vi "get_config_multiplex.vi"(10 "target R":dbl format="%#_13g", 11 "configs":cluster{"R":dbl, "relays":bool[]}[](array[cluster])) -> (2 "index":i32, 3 "multiplexor":bool[](array[boolean]))   [LabVIEW 2018]
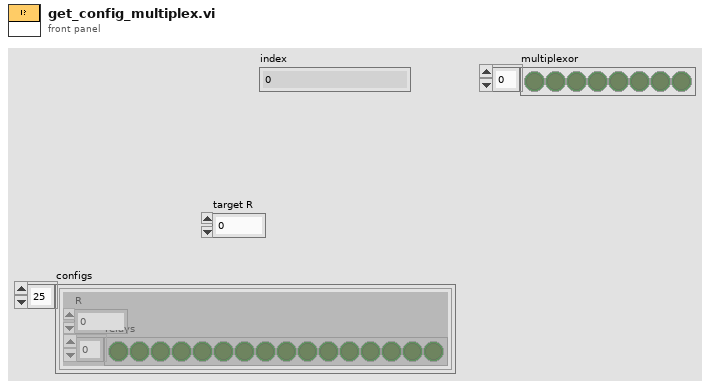
[diagram p1: front panel]
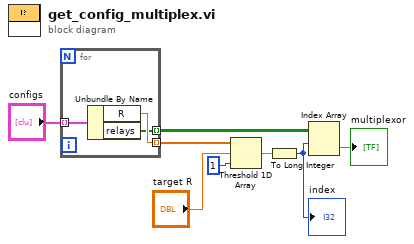
[diagram p0: block diagram]
diagram:
  n1 = for {
    tunnel: "configs" -> [w11] mode=indexing
    tunnel: [w10] -> w2 mode=indexing
    tunnel: [w9] -> w1 mode=indexing
    n2 = Unbundle By Name(w11) -> ("R"=w10:dbl, "relays"=w9:bool[])
  }
  n3 = Threshold 1D Array(1:1 ("indice de départ (0)"), 2:"target R", 3:w2) -> (0:w7:dbl)
  n4 = To Long Integer(number=w7) -> (32bit integer=w5:i32)
  "index" <- w5
  n5 = Index Array(array=w1, index (row)=w5) -> (element=→"multiplexor":bool[])  [unwired: 1 in]
